vi "reset sesion.vi"(8 "error in (no error)":errorcluster, 11 "USRP_1_x_200MHz in":refnum<class "USRP_1_x_200MHz.lvclass">) -> (0 "error out":errorcluster, 3 "USRP_1_x_200MHz out":refnum<class "USRP_1_x_200MHz.lvclass">)   [LabVIEW 2021, in "USRP_1_x_200MHz.lvclass"]
uses:
  USRP_1_x_200MHz.lvclass
  USRP_1_x_200MHz.lvclass/USRP_1_x_200MHz.ctl
  <vilib>/Utility/error.llb/Error Cluster From Error Code.vi
  <vilib>/rvi/errors/niLvFpgaAdjustHostInterfaceError.vi
  <vilib>/rvi/interface/nirviReadWriteControl/nirviReadWriteControl.xnode
  <vilib>/rvi/interface/nirviMethod/nirviMethod.xnode
  NiFpgaLv.dll
  <vilib>/rvi/interface/Simulation/niFpgaSimulationCallBeginRW.vi
  <vilib>/FPGAPlugInAG/Dynamic/niLvFpga_StopFifo_Dynamic.vi
  <vilib>/rvi/errors/niLvFpgaMergeErrorWithErrorCode.vi
  <vilib>/FPGAPlugInAG/Dynamic/niLvFpga_StartFifo_Dynamic.vi
panel:
  out "debug mode 2":T1
  out "debug mode":T1
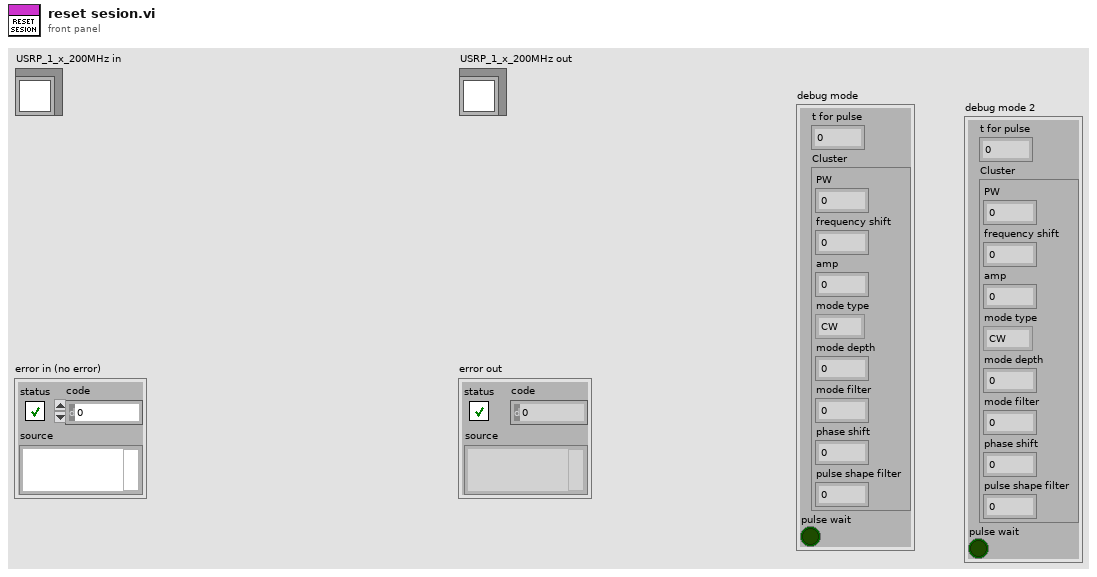
[diagram p1: front panel]
types:
  T1 = cluster{"t for pulse":u64, "Cluster":cluster{"PW":u32, "frequency shift":fxp<+/-,48,0>, "amp":fxp<+/-,18,1>, "mode type":enum8{"CW", "from memory 1", "NC - cw", "LFM", "BPSK", "QPSK"}, "mode depth":u32, "mode filter":u8, "phase shift":fxp<+/-,16,1>, "pulse shape filter":u8}, "pulse wait":bool}
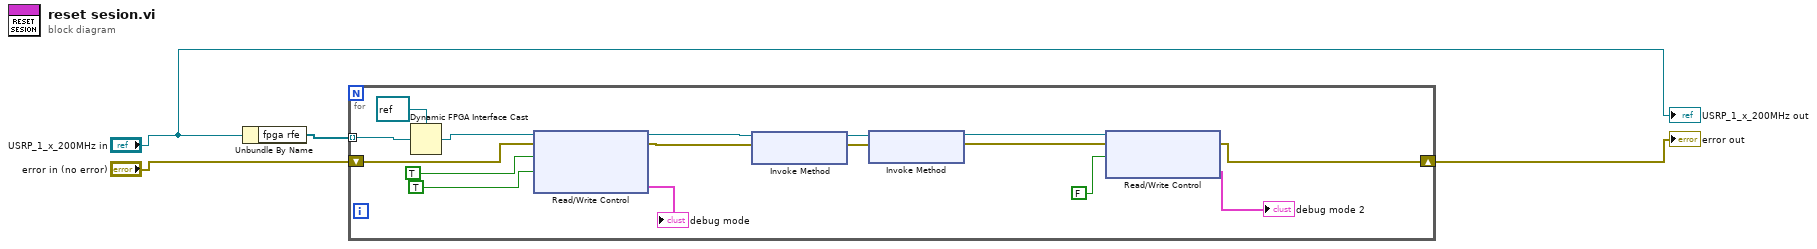
[diagram p0: block diagram]
diagram:
  n1 = Unbundle By Name("USRP_1_x_200MHz in") -> ("fpga rfe"=w4:refnum<k20>[])
  n2 = for {
    tunnel: w4 -> [w18] mode=indexing
    shift-right: [w14] -> w3
    shift-left: "error in (no error)" -> [w19]
    n3 = Dynamic FPGA Interface Cast(Session In=refnum<k20> refnum ("FPGA VI Reference Out"), Type=w18) -> (Session Out=w17:refnum<k20>)
    n4 = xnode "Read/Write Control"("FPGA VI Reference In"=w17, "error in"=w19, "reset system clock"=TRUE, "IQ_run"=TRUE) -> ("FPGA VI Reference Out"=w10:refnum<k20>, "error out"=w9:errorcluster, "debug mode"=→"debug mode":T1)
    n5 = xnode "Invoke Method"("FPGA VI Reference In"=w10, "error in"=w9) -> ("FPGA VI Reference Out"=w8:refnum<k20>, "error out"=w7:errorcluster)
    n6 = xnode "Invoke Method"("FPGA VI Reference In"=w8, "error in"=w7) -> ("FPGA VI Reference Out"=w5:refnum<k20>, "error out"=w6:errorcluster)
    n7 = xnode "Read/Write Control"("FPGA VI Reference In"=w5, "error in"=w6, "reset system clock"=FALSE) -> ("error out"=w14:errorcluster, "debug mode"=→"debug mode 2":T1)  [unwired: 1 out]
  }
  "error out" <- w3
  "USRP_1_x_200MHz out" <- "USRP_1_x_200MHz in"
